vi "util-analog-filter.vi"(10 "Array":dbl[](array[numeric]), 11 "# of mins&maxs to remove":i32) -> (2 "Filtered Value":dbl)   [LabVIEW 2024]
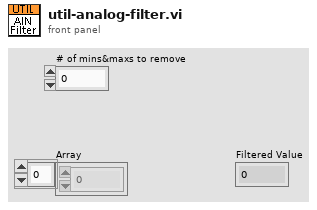
[diagram p1: front panel]
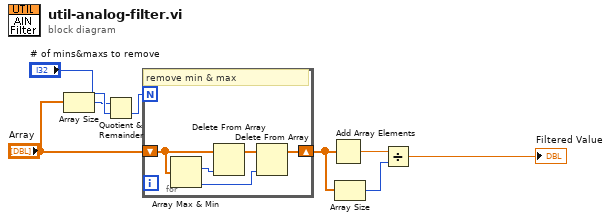
[diagram p0: block diagram]
diagram:
  n1 = Array Size(array="Array") -> (size(s)=w6:i32)
  n2 = Quotient & Remainder(x=w6, y="# of mins&maxs to remove") -> (floor(x/y)=w8:i32)  [unwired: 1 out]
  n3 = for {
    N: w8 -> [_]
    shift-right: [w10] -> w3
    shift-left: "Array" -> [w13]
    # "remove min & max"
    n4 = Array Max & Min(array=w13) -> (max index (indices)=w12:i32, min index (indices)=w9:i32)  [unwired: 2 out]
    n5 = Delete From Array(array=w13, index=w12) -> (array with subset deleted=w11:dbl[])  [unwired: 1 in, 1 out]
    n6 = Delete From Array(array=w11, index=w9) -> (array with subset deleted=w10:dbl[])  [unwired: 1 in, 1 out]
  }
  n7 = Add Array Elements(numeric array=w3) -> (sum=w1:dbl)
  n8 = Array Size(array=w3) -> (size(s)=w2:i32)
  n9 = Divide(x=w1, y=w2) -> (x/y=→"Filtered Value":dbl)
